vi "Finish.vi"   [LabVIEW 2018]
doc: "This VI is called just before exiting. It is expected to close I/O refnum, save collected data, etc."
uses:
  RobotGlobal.vi
  Classes/Pnematics control/Pneumatics.lvclass
  Classes/Drive/Drive.lvclass
  Classes/Vision/Vision.lvclass
  Classes/Cargo/Cargo.lvclass
  Classes/Joysticks/Joysticks.lvclass
  Classes/Hatch/Hatch.lvclass
  Classes/Elevator/Elevator.lvclass
types:
  T1 = typedef "RobotObjects.ctl" = cluster{"Drive.lvclass":refnum<class "Drive.lvclass">, "Pneumatics.lvclass":refnum<class "Pneumatics.lvclass">, "Vision.lvclass":refnum<class "Vision.lvclass">, "Joysticks.lvclass":refnum<class "Joysticks.lvclass">, "Elevator.lvclass":refnum<class "Elevator.lvclass">, "Hatch.lvclass":refnum<class "Hatch.lvclass">, "Cargo.lvclass":refnum<class "Cargo.lvclass">}
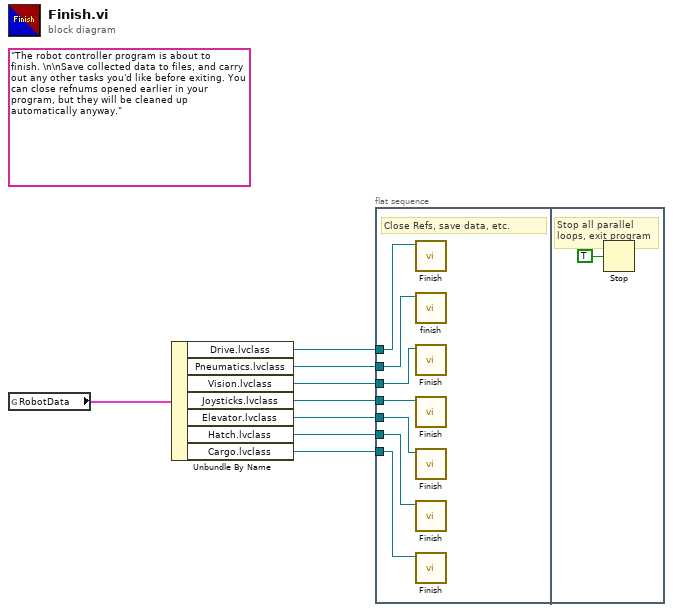
[diagram p0: block diagram]
diagram:
  (unwired) "The robot controller program is about to finish. \n\nSave collected data to files, and carry out any other tasks you'd like before exiting. You can close refnums opened earlier in your program, but they will be cleaned up automatically anyway."
  n1 = global read "RobotGlobal.vi" "RobotData"() -> (w8:T1)
  n2 = Unbundle By Name(w8) -> ("Drive.lvclass"=w6:refnum<class "Drive.lvclass">, "Pneumatics.lvclass"=w7:refnum<class "Pneumatics.lvclass">, "Vision.lvclass"=w5:refnum<class "Vision.lvclass">, "Joysticks.lvclass"=w3:refnum<class "Joysticks.lvclass">, "Elevator.lvclass"=w1:refnum<class "Elevator.lvclass">, "Hatch.lvclass"=w2:refnum<class "Hatch.lvclass">, "Cargo.lvclass"=w4:refnum<class "Cargo.lvclass">)
  n3 = flat-sequence {
    tunnel: w7 -> [w15]
    tunnel: w6 -> [w14]
    tunnel: w5 -> [w13]
    tunnel: w4 -> [w12]
    tunnel: w3 -> [w11]
    tunnel: w2 -> [w10]
    tunnel: w1 -> [w9]
    frame #0 {
      # "Close Refs, save data, etc."
      n4 = call-dynamic "Finish.vi"("Drive in"=w14) -> ()  [unwired: 9 in, 2 out]
      n5 = call-dynamic "finish.vi"("Pneumatics in"=w15) -> ()  [unwired: 9 in, 2 out]
      n6 = call-dynamic "Finish.vi"("Vision in"=w13) -> ()  [unwired: 9 in, 2 out]
      n7 = call-dynamic "Finish.vi"("Joysticks in"=w11) -> ()  [unwired: 9 in, 2 out]
      n8 = call-dynamic "Finish.vi"("Elevator in"=w9) -> ()  [unwired: 9 in, 2 out]
      n9 = call-dynamic "Finish.vi"("Hatch in"=w10) -> ()  [unwired: 9 in, 2 out]
      n10 = call-dynamic "Finish.vi"("Cargo in"=w12) -> ()  [unwired: 9 in, 2 out]
    }
    frame #1 {
      # "Stop all parallel\nloops, exit program"
      n11 = Stop(stop? (T)=TRUE ("Quit")) -> ()
    }
  }
